vi "Q Ref FGV.vi"(7 "Command":T1, 8 "error in (no error)":errorcluster) -> (0 "error out":errorcluster, 3 "Q Ref":refnum<queue>)   [LabVIEW 2010, in "Template Module.lvlib"]
uses:
  Template Module.lvlib
  Q Message Cluster.ctl
  Q Ref FGV Command Enum.ctl
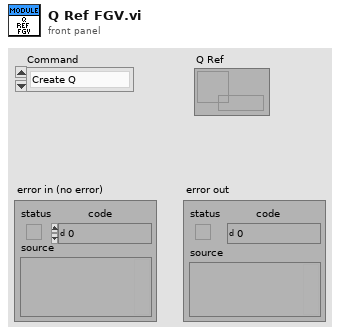
[diagram p1: front panel]
types:
  T1 = typedef "Template Module.lvlib/Q Ref FGV Command Enum.ctl" = enum16{"Create Q", "Get Q", "Flush Q", "Release Q"}
  T2 = typedef "Template Module.lvlib/Q Message Cluster.ctl" = cluster{"Message":string, "Data":variant}
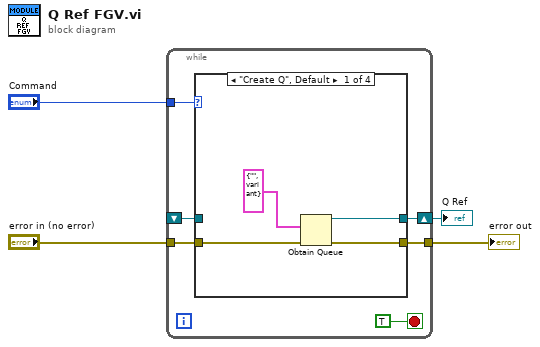
[diagram p0: block diagram]
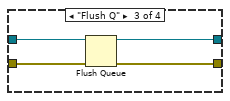
[diagram p3: hidden frame]
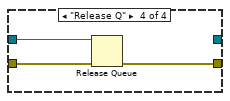
[diagram p4: hidden frame]
diagram:
  n1 = while {
    tunnel: "Command" -> [w9]
    shift-right: [w8] -> w2
    shift-left: _ -> [w7]
    tunnel: [w6] -> w3
    tunnel: "error in (no error)" -> [w5]
    stop <- TRUE stop-if-true
    n2 = case shown="\"Create Q\", Default" w9 {
      tunnel: [w13 w16 w17 _] -> w8
      tunnel: w7 -> [_ w16 w20 w21]
      tunnel: [w12 w15 w18 w22] -> w6
      tunnel: w5 -> [w11 w15 w19 w23]
      frame "Create Q", Default {
        n3 = Obtain Queue(element data type=T2 {"Message"="", "Data"=variant} ("Q Message Cluster"), error in (no error)=w11) -> (queue out=w13:refnum<queue>, error out=w12:errorcluster)  [unwired: 3 in, 1 out]
      }
      frame "Get Q" {
      }
      frame "Flush Q" {
        n4 = Flush Queue(queue=w20, error in (no error)=w19) -> (queue out=w17:refnum<queue>, error out=w18:errorcluster)  [unwired: 1 out]
      }
      frame "Release Q" {
        n5 = Release Queue(queue=w21, error in (no error)=w23) -> (error out=w22:errorcluster)  [unwired: 1 in, 2 out]
      }
    }
  }
  "error out" <- w3
  "Q Ref" <- w2
